vi "swmm_start.vi"(3 "error in (no error)":errorcluster, 4 "Success msg?":bool, 5 "Write Report?":bool) -> (0 "error out":errorcluster)   [LabVIEW 2014]
uses:
  swmm5.dll
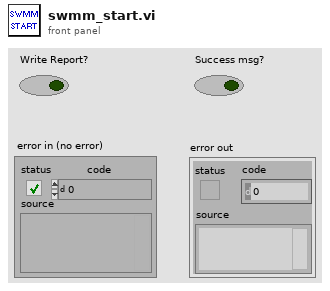
[diagram p1: front panel]
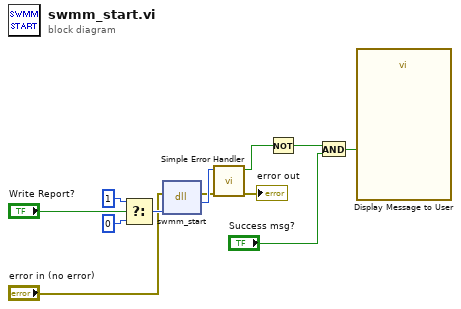
[diagram p0: block diagram]
diagram:
  n1 = Select(t=1, s="Write Report?", f=0) -> (s? t:f=w9:i32)
  n2 = dll-call lib="PTH2zabs CUsers\nandres riañoDropboxProyecto AguasSoftwareMatSWMMMatSWMM 5.1.009LabVIEW modulex64\tswmm5.dll" fn="swmm_start"(error in="error in (no error)", "write_report"=w9) -> (error out=w7:errorcluster, "return type"=w8:i32)  [unwired: 3 in, 1 out]
  n3 = call <vilib>:"Simple Error Handler.vi"("error code (no error:0)"=w8, "error in (no error)"=w7) -> ("error?"=w3:bool, "error out"=→"error out":errorcluster)  [unwired: 3 in, 3 out]
  n4 = Not(x=w3) -> (.not. x?=w6:bool)
  n5 = And(x=w6, y="Success msg?") -> (x .and. y?=w4:bool)
  n6 = call "Display Message to User"("Enable"=w4) -> ()  [unwired: 9 in, 2 out]
